vi "Quadratic JTFA Method.vi"() -> ()   [LabVIEW 2023]
doc: "This example shows the signal processing procedure of quadratic TFA methods. In practice, the procedure includes the following steps:\n\n1) Compute the spectrogram of a signal, such as STFT spectrogram, Gabor spectrogram, adaptive spectrogram, and so on.\n2) Extract features from the spectrogram, such as instantaneous frequency, group delay, and so on.\n3) Perform pattern recognition and make decisions based on the extracted features and the spectrogram.\n\n<b>Instructions:</b>\nRun this VI to understand the flowchart of quadratic TFA applications."
uses:
  <vilib>/addons/Time Frequency Analysis/typedefs.llb/TFA Data.ctl
  Instance           4 29Saved   Quadratic JTFA Method .vi
  <vilib>/addons/Time Frequency Analysis/_control.llb/TFA Configure Spectrogram Indicator (Predefined Color Table).vi
  <vilib>/addons/_Advanced Signal Processing/NI_AdvSigProcTFA.lvlib
panel:
  out "aspt-left-top":bool
  out "Spectrogram":dbl[][](graph)
  out "Mean Instantaneous Frequency":cluster{"t0":dbl, "dt":dbl, "frequency":dbl[]}(graph)
  out "Source Signal":waveform(dbl)(graph)
  # "Overview: Shows the signal processing procedure of quadratic TFA methods.\nRequirements: LabVIEW Full Development System, Advanced Signal Processing Toolkit\nInstructions: \nRun this VI to understand the flowchart of quadratic TFA applications."
  # "Pattern Recognition\n& Decision Making"
  # "2D result"
  # "1D result"
  # "Feature Extraction"
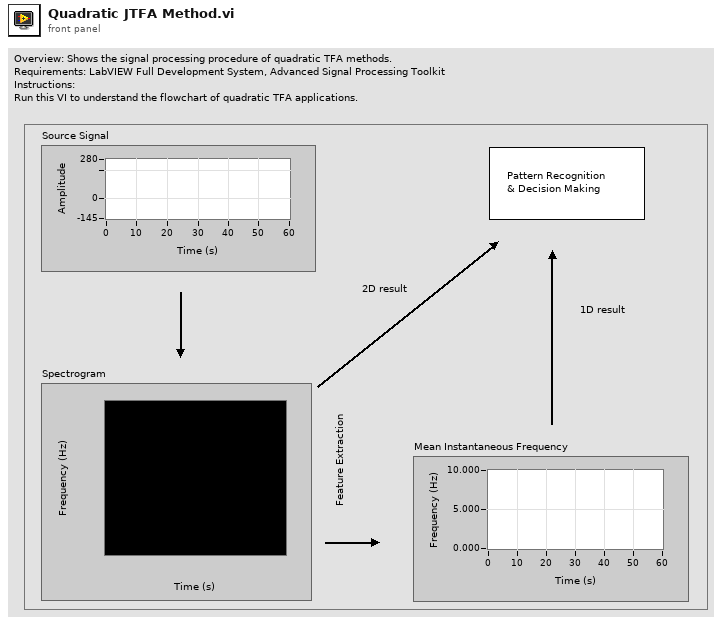
[diagram p1: front panel]
types:
  T1 = typedef "NI_AdvSigProcTFA.lvlib/TFA Data.ctl" = u16
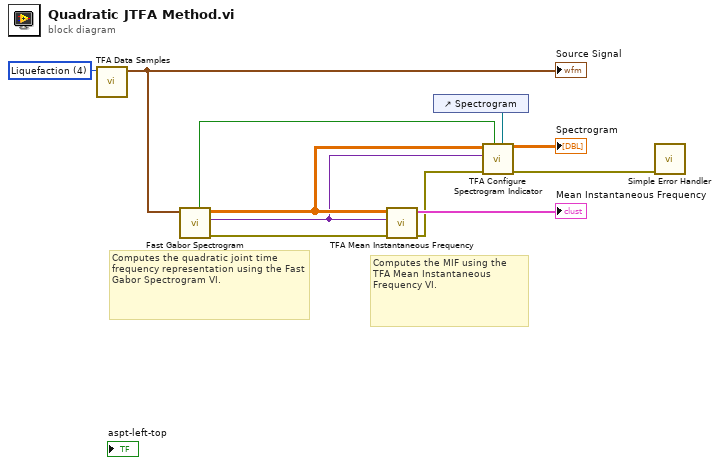
[diagram p0: block diagram]
diagram:
  w4 = T1 4 items=["PC Fan"=0, "Noisy Chirps"=1, "TDR 1"=2, "TDR 2"=3, "Liquefaction"=4, "Liquefaction Free"=5, "Aneurysm"=6, "Bat"=7, "RF"=8, "Two Gaussian"=9, "Three Gaussian"=10, "Chirp"=11, "Gaussian Chirp"=12, "Cross Chirp"=13, "Doppler"=14, "HOP"=15, "TF Sine"=16, "Three Tone"=17, "Four Tone"=23, "Blood Flow Doppler (phase a)"=20, "Blood Flow Doppler (phase b)"=21, "Heart sound"=22, "-"=18, "Random Noise"=19] ("data")
  # "Computes the quadratic joint time frequency representation using the Fast Gabor Spectrogram VI."
  # "Computes the MIF using the TFA Mean Instantaneous Frequency VI."
  n1 = call <vilib>:"TFA Data Samples.vi"("data"=w4) -> ("signal"=w8:waveform(dbl))  [unwired: 10 out]
  "Source Signal" <- w8
  n2 = call "Fast Gabor Spectrogram"("Signal"=w8) -> ("error out"=w3:errorcluster, "Scale Info"=w5:variant, "Spectrogram"=w6:dbl[][], "dB"=w7:bool)  [unwired: 2 in, 5 out]
  n3 = call <vilib>:"TFA Mean Instantaneous Frequency.vi"("error in (no error)"=w3, "scale info"=w5, "spectrogram"=w6) -> ("error out"=w2:errorcluster, "MIF"=→"Mean Instantaneous Frequency":cluster{"t0":dbl, "dt":dbl, "frequency":dbl[]})  [unwired: 7 out]
  n4 = control-ref of="Spectrogram"() -> (w10:refnum<vi>)
  n5 = call-poly <vilib>:"TFA Configure Spectrogram Indicator.vi"("reference of TF spectrogram indicator"=w10, "dB on? (F)"=w7, "error in (no error)"=w2, "scale info"=w5, "spectrogram"=w6) -> ("error out"=w1:errorcluster, "TF spectrogram indicator"=→"Spectrogram":dbl[][])  [unwired: 2 in, 3 out]
  n6 = call <vilib>:"Simple Error Handler.vi"("error in (no error)"=w1) -> ()  [unwired: 4 in, 5 out]
